vi "Dialog.vi"() -> ()   [LabVIEW 2014]
panel:
  in  "OK Button":bool
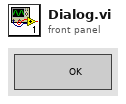
[diagram p1: front panel]
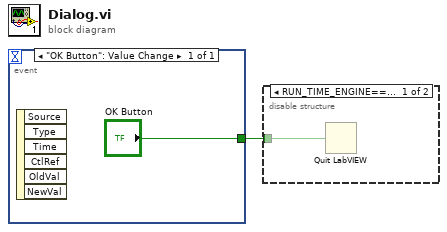
[diagram p0: block diagram]
diagram:
  n1 = event shown="[0] \"OK Button\": Value Change" {
    selector: _ -> [_]
    dyn-events: _ -> [_]
    timeout: _ -> [_]
    tunnel: ["OK Button"] -> w1
    event "OK Button": Value Change {
      n2 = event-data() -> ()  [unwired: 1 in, 6 out]
    }
  }
  n3 = disable-structure shown="RUN_TIME_ENGINE==True" {
    disable-tunnel: w1 -> [w3 _]
    frame condition #0 {
      n4 = Quit LabVIEW(quit? (T)=w3) -> ()
    }
    frame condition #1 (active) {
    }
  }
